vi "Read.vi"(8 "error in (no error)":errorcluster, 9 "max bytes to read":i32 min=0 max=65535, 10 "core reader handle in":u64, 11 "core handle in":u64) -> (0 "error out":errorcluster, 1 "bytes read":i32, 2 "core reader handle out":u64, 3 "core handle out":u64)   [LabVIEW 2020, in "Ballard ARINC 429 Hardware API.lvlib"]
doc: "Reads sequential records associated with <B>core handle in</B> into the <B>reader handle in</B> object. <B>max bytes to read</B> is capped at 65,535.\n\nThis VI will fail if the configuration file's <B>sequentialLog.perChannelStreaming</B> is true. If the configuration file's <B>sequentialLog</B> node is not defined for this device, this function will always read 0 records.\n\nIf you are not seeing records like you would expect, several things must be verified to ensure the device has been setup for recording the way you want:\n1. Ensure you have already called a Configure VI for the device and channels you desire to record.\n2. Ensure you have not stopped the sequential monitor with the <B>Stop Sequential Monitor</B> VI.\n3. Verify the configuration file has defined the <B>sequentialLog</B> node.\n4. Verify the configuration file has not been set-up to filter out or disable monitoring on the channel or messages you are wanting to record. See the BTI1553LV and BTI429LV libraries for more information on protocol-specific filtering options in the configuration file."
uses:
  Ballard ARINC 429 Hardware API.lvlib
  BTICardLV.dll
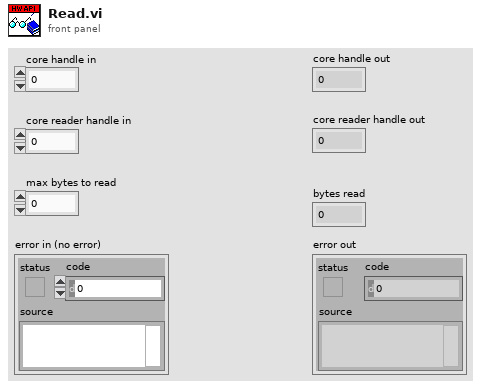
[diagram p1: front panel]
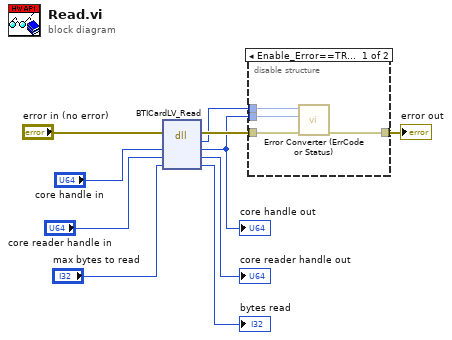
[diagram p0: block diagram]
diagram:
  n1 = dll-call lib="BTICardLV.*" fn="BTICardLV_Read"(error in="error in (no error)", "corehandle"="core handle in", "readerhandle"="core reader handle in", "bytes"="max bytes to read") -> (error out=w5:errorcluster, "return type"=w3:i32, "corehandle"=w2:u64, "readerhandle"=→"core reader handle out":u64, "bytes"=→"bytes read":i32)  [unwired: 2 in, 1 out]
  "core handle out" <- w2
  n2 = disable-structure shown="Enable_Error==TRUE" {
    disable-tunnel: w5 -> [w14 w15]
    disable-tunnel: [w13 w15] -> w4
    disable-tunnel: w3 -> [w12 _]
    disable-tunnel: w2 -> [w11 _]
    frame condition #0 {
      n3 = call "Error Converter (ErrCode or Status).vi"("error in (no error)"=w14, "handle in"=w11, "error code"=w12) -> ("error out"=w13:errorcluster)  [unwired: 8 in]
    }
    frame condition #1 (active) {
    }
  }
  "error out" <- w4
